vi "Total Data.vi"(10 "Contol\nPoint\nSuffix":T1, 11 "Cartesian Type":bool) -> (3 "Data":dbl[](array[numeric]))   [LabVIEW 2009]
uses:
  NTCP Client/Control Point Suffix.ctl
  Actuator Measurment Actions.ctl
  Cartesian Measurment Actions.ctl
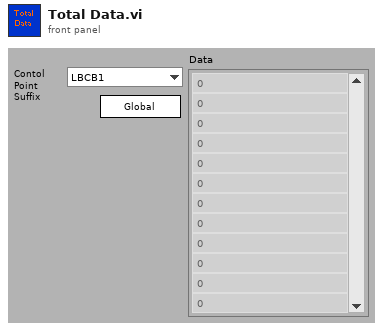
[diagram p1: front panel]
types:
  T1 = typedef "Control Point Suffix.ctl" = enum16{"LBCB1", "LBCB2", "ExternalSensors"}
  T2 = typedef "Cartesian Measurment Actions.ctl" = enum16{"Set Data", "Get", "Init", "Set Offsets"}
  T3 = typedef "Actuator Measurment Actions.ctl" = enum16{"Set  Data", "Get", "Init"}
  T4 = typedef "LBCB Number.ctl" = enum16{"LBCB1", "LBCB2"}
  T5 = typedef "Actuator DataType.ctl" = cluster{"LVDTs":dbl[], " Commands":dbl[], "Load Cells":dbl[], "Servo":dbl[]}
  T6 = typedef "Cartesian Data Type.ctl" = cluster{"Displacements":dbl[], "Forces":dbl[], "Displacement Commands":dbl[]}
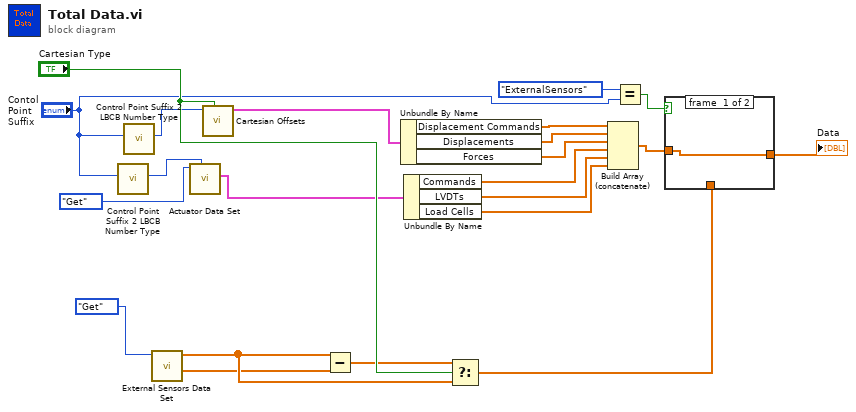
[diagram p0: block diagram]
diagram:
  n1 = call "Control Point Suffix 2 LBCB Number Type.vi"("Contol\nPoint\nSuffix"="Contol\nPoint\nSuffix") -> ("LBCB Number"=w5:T4)  [unwired: 10 out]
  n2 = call "Control Point Suffix 2 LBCB Number Type.vi"("Contol\nPoint\nSuffix"="Contol\nPoint\nSuffix") -> ("LBCB Number"=w11:T4)  [unwired: 10 out]
  n3 = call "External Sensors Data Set.vi"("Measurement Actions"=Cartesian_Measurment_Actions."Get") -> ("Offsets"=w2:dbl[], "External Sensors Out"=w3:dbl[])  [unwired: 3 in, 6 out]
  n4 = call "Actuator Data Set.vi"("Selected LBCB"=w5, "Measurement Actions"=Actuator_Measurment_Actions."Get") -> ("Actuator Data Out"=w4:T5)  [unwired: 3 in, 6 out]
  n5 = call "Cartesian Offsets.vi"("Use Offsets"="Cartesian Type", "LBCB Number"=w11) -> ("Cartesian Data Out"=w7:T6)  [unwired: 7 out]
  n6 = Subtract(x=w3, y=w2) -> (x-y=w1:dbl[])
  n7 = Unbundle By Name(w7) -> ("Displacement Commands"=w21:dbl[], "Displacements"=w20:dbl[], "Forces"=w19:dbl[])
  n8 = Unbundle By Name(w4) -> ("Commands"=w18:dbl[], "LVDTs"=w17:dbl[], "Load Cells"=w16:dbl[])
  n9 = Select(t=w1, s="Cartesian Type", f=w3) -> (s? t:f=w12:dbl[])
  n10 = Build Array (concatenate)(w21, w20, w19, w18, w17, w16) -> (w15:dbl[])
  n11 = Equal?(x=Control_Point_Suffix."ExternalSensors", y="Contol\nPoint\nSuffix") -> (x = y?=w10:bool)
  n12 = case shown="True" w10 {
    tunnel: w15 -> [w23 _]
    tunnel: [w23 w24] -> w13
    tunnel: w12 -> [_ w24]
    frame #0 {
    }
    frame #1 {
    }
  }
  "Data" <- w13
